vi "Current Limiter.vi"() -> (3 "CurrentOK":bool=TRUE)   [LabVIEW 2015]
uses:
  Global Data.vi
panel:
  in  "% Fuse":i32
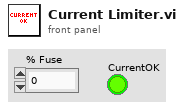
[diagram p1: front panel]
types:
  T1 = typedef "FPGA Telemetry.ctl" = cluster{"CPU Load":cluster{"Total (%)":dbl, "Time Critical (%)":dbl, "Timed Structures (%)":dbl, "High (%)":dbl, "Above Normal (%)":dbl, "Normal (%)":dbl, "Background (%)":dbl, "Idle (%)":dbl, "ISR (%)":dbl}, "SVehicleStatus":cluster{"BMS Status":T2, "MC Status":T2, "Shutdown Status":T2, "sbRIO Status":T2, "Vehicle Status":T2, "Shutdown State":enum16{"NI.SC.Initial", "NI.SC.History", "NI.SC.ShallowHistory", "NI.SC.Terminal", "Coolant Pump Started/AIR's On", "AIRs On", "Precharge", "TSMS Off"}, "AIR Status":T5, "Remote Return to Pits":bool, "Reason for Shutdown":T6, "MC State Machine Status":enum16{"NI.SC.Initial", "NI.SC.History", "NI.SC.ShallowHistory", "NI.SC.Terminal", "Broadcast Diag", "Let Current Drop then Disable AIR's", "Enabled", "Disabled"}}, "iPhone HF Data":cluster{"gXiPhone":dbl, "gYiPhone":dbl, "gZiPhone":dbl, "nYawXiPhone":dbl, "nYawYiPhone":dbl, "nYawZiPhone":dbl}, "iPhone LF Data":cluster{"nLatiPhone":dbl, "nLongiPhone":dbl, "nGPSiPhone":dbl}, "stop":bool, "VSupplyOffset":fxp<+,12,4>, "VsbRIOSupply":fxp<+/-,25,6>, "bFPGALED":bool, "TSBRIO":fxp<+/-,33,17>, "rTPS2Unscaled":fxp<+/-,16,1>, "rTPS1Unscaled":fxp<+/-,16,1>, "bTPSConsistent":bool, "bTPSInRange":bool, "rThrottle":fxp<+/-,33,22>, "VTPS2":fxp<+/-,24,5>, "rTPS2":fxp<+/-,31,22>, "VTPS1":fxp<+/-,24,5>, "rTPS1":fxp<+/-,31,22>, "rTPS2Max":fxp<+,16,4>, "rTPS2Min":fxp<+,16,4>, "rTPS1Max":fxp<+,16,4>, "rTPS1Min":fxp<+,16,4>, "bCoolantPumpEnable":bool, "bRTDSEnable":bool, "bTSMSInStatus":bool, "bPosAIREnable":bool, "bBMSOK":bool, "bIMDOK":bool, "bBSPDOK":bool, "bSBRIOOK2":bool, "bSBRIOOK1":bool, "bTSMSOutStatus":bool, "eGreenDash":T7, "eYellowDash":T7, "eRedDash":T7, "bMotorControllerEnable":bool, "tCurrentLap":u32, "bNewLap":bool, "tLastLap":u32, "tLapMin":u32, "V5VSupply":fxp<+/-,24,5>, "bWheelRL":bool, "bWheelRR":bool, "bWheelFR":bool, "bWheelFL":bool, "VBrakePressureR":fxp<+/-,24,5>, "VBrakePressureF":fxp<+/-,24,5>, "bWheelRRStopped":bool, "bWheelRLStopped":bool, "bWheelFRStopped":bool, "bWheelFLStopped":bool, "tWheelRLPeriod":u32, "tWheelRRPeriod":u32, "tWheelFRPeriod":u32, "tWheelFLPeriod":u32, "bBrakeLight":bool, "VShockRR":fxp<+/-,24,5>, "VShockRL":fxp<+/-,24,5>, "VShockFR":fxp<+/-,24,5>, "VShockFL":fxp<+/-,24,5>, "IHighCurrent":fxp<+/-,24,15>, "ILowCurrent":fxp<+/-,24,15>, "pBrakeR":fxp<+,26,13>, "pBrakeF":fxp<+,26,13>, "bHighCurrentOK":bool, "bLowCurrentOK":bool, "bBrakeROK":bool, "bBrakeFOK":bool, "VSteerWheelMiddle":fxp<+/-,26,5>, "aSteerWheel":fxp<+/-,31,13>, "nWheelFL":fxp<+/-,32,16>, "nWheelFR":fxp<+/-,32,16>, "nWheelRL":fxp<+/-,32,16>, "nWheelRR":fxp<+/-,32,16>, "ADXL345 Output":T8, "Tire Diameter(m)":fxp<+,16,1>, "vWheelRR":fxp<+/-,32,18>, "vWheelRL":fxp<+/-,32,18>, "vWheelFR":fxp<+/-,32,18>, "vWheelFL":fxp<+/-,32,18>, "vWheelLowest":fxp<+/-,32,18>, "vWheelHighest":fxp<+/-,32,18>, "bAccel":bool, "vAxleF":fxp<+/-,33,19>, "vCar":fxp<+/-,33,19>, "sLap":fxp<+,32,12>, "rSlipRL":fxp<+/-,12,1>, "rSlipRR":fxp<+/-,12,1>, "rSlipFL":fxp<+/-,12,1>, "rSlipFR":fxp<+/-,12,1>, "NLap":u8, "tLapReference":u32, "tFastestLap":u32, "MTorqueRequest":dbl, "RS232 Error Out":cluster{"status":bool, "code":i32}}
  T2 = typedef "Subsystem Status.ctl" = cluster{"eStatusSeverity":T3, "NValue":sgl, "CMessage":T4, "bNotOK":bool}
  T3 = typedef "Subsystem Status Severity.ctl" = enum16{"Okay", "Short Warning", "Long Warning", "Return to Pits", "Error", "Danger"}
  T4 = typedef "Subsystem Status Message.ctl" = enum16{"ControllerTemperature", "MotorTemperature", "BatteryTemperature", "BatteryLowVoltage", "LVBattery", "sbRIOTemperature", "Precharge", "BSPD", "IMD", "RemoteReturnToPits", "EStopInterrupted", "NoCellComms", "MCOverSpeed", "MCOverCurrent", "MCOverVoltage", "MCInverterOverTemp", "MCDirectionCommand", "MCInverterTimeout", "MCDesatFault", "MCHWOverCurrent", "MCUnderVoltage", "MCCommandMessageLost", "MotorOverTemp", "MCModAOverTemp", "MCModBOverTemp", "MCModCOverTemp", "MCPCBOverTemp", "MCGateDrv1OverTemp", "MCDateDrv2OverTemp", "MCCurrentSensorFault", "MCResolverNotConnected", "ShutdownLatchTripped", "UnknownBMS", "RemoteEmergency"}
  T5 = typedef "AIR Status.ctl" = enum16{"Off", "Precharge", "On"}
  T6 = typedef "Reason for Shutdown.ctl" = enum16{"None", "BMS", "Shutdown", "sbRIO", "MC", "Remote"}
  T7 = typedef "Dash LED Status.ctl" = enum16{"Off", "Flashing", "On"}
  T8 = typedef "ADXL345 Output.ctl" = cluster{"X":fxp<+/-,14,4>, "Y":fxp<+/-,14,4>, "Z":fxp<+/-,14,4>}
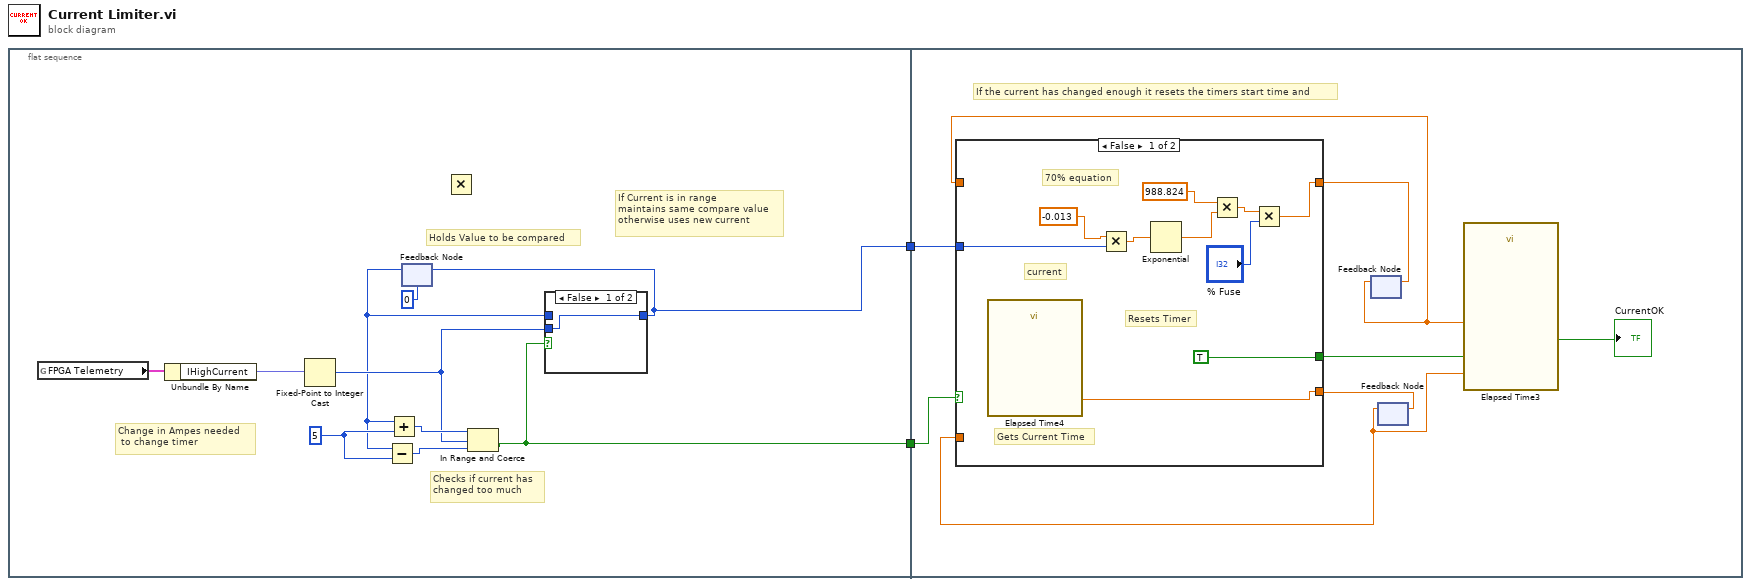
[diagram p0: block diagram]
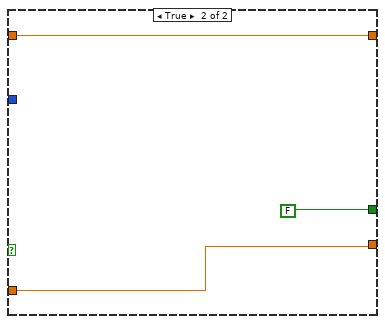
[diagram p3: hidden frame]
diagram:
  n1 = flat-sequence {
    tunnel: [w4] -> w2
    tunnel: [w3] -> w1
    tunnel: w2 -> [w22]
    tunnel: w1 -> [w18]
    frame #0 {
      w10 = 5
      # "Checks if current has\nchanged too much"
      # "If Current is in range\nmaintains same compare value\notherwise uses new current"
      # "Holds Value to be compared"
      # "Change in Ampes needed\n to change timer"
      n2 = global read "Global Data.vi" "FPGA Telemetry"() -> (w12:T1)
      n3 = Unbundle By Name(w12) -> ("IHighCurrent"=w11:fxp<+/-,24,15>)
      n4 = Fixed-Point to Integer Cast(1:w11) -> (0:w6:i32)
      n5 = feedback #1(0) -> (w5:i32)
      n6 = Subtract(x=w5, y=w10) -> (x-y=w9:i32)
      n7 = Add(x=w5, y=w10) -> (x+y=w8:i32)
      n8 = Multiply() -> ()  [unwired: 2 in, 1 out]
      n9 = In Range and Coerce(upper limit=w8, x=w6, lower limit=w9) -> (In Range?=w4:bool)  [unwired: 1 out]
      n10 = case shown="False" w4 {
        tunnel: w6 -> [w13 _]
        tunnel: w5 -> [_ w14]
        tunnel: [w13 w14] -> w3
        frame False {
        }
        frame True {
        }
      }
      n11 = feedback-in #1(w3) -> ()
    }
    frame #1 {
      # "If the current has changed enough it resets the timers start time and"
      n12 = feedback #2() -> (w16:dbl)  [unwired: 1 in]
      n13 = feedback #3() -> (w19:dbl)  [unwired: 1 in]
      n14 = case shown="False" w22 {
        tunnel: [w31 w34] -> w21
        tunnel: [TRUE FALSE] -> w20
        tunnel: w19 -> [_ w34]
        tunnel: w18 -> [w26 _]
        tunnel: [w23 w33] -> w17
        tunnel: w16 -> [_ w33]
        frame False {
          # "Gets Current Time"
          # "current"
          # "70% equation"
          # "Resets Timer"
          n15 = call "Elapsed Time4"() -> ("Present (s)"=w31:dbl)  [unwired: 12 in, 7 out]
          n16 = Multiply(x=-0.013, y=w26) -> (x*y=w29:dbl)
          n17 = Exponential(1:w29) -> (0:w28:dbl)
          n18 = Multiply(x=988.824, y=w28) -> (x*y=w25:dbl)
          n19 = Multiply(x=w25, y="% Fuse") -> (x*y=w23:dbl)
        }
        frame True {
        }
      }
      n20 = feedback-in #2(w17) -> ()
      n21 = feedback-in #3(w21) -> ()
      n22 = call "Elapsed Time3"("Time Target (s)"=w16, "Reset"=w20, "Set Start Time (s)"=w19) -> ("Time has Elapsed"=→"CurrentOK":bool)  [unwired: 9 in, 7 out]
    }
  }
